vi "GetDigital.vi"(0 "reference in":refnum<class "Digital.lvclass">, 5 "error in (no error)":errorcluster) -> (14 "reference out":refnum<class "Digital.lvclass">, 19 "error out":errorcluster)   [LabVIEW 2019, in "Digital.lvclass"]
doc: "Draws A button"
uses:
  Digital.lvclass
  C:/Users/Taylor.Hillegeist/OneDrive - Ultra/LabVIEW/Pgui2/Pgui_Obj_class/Pgui_Obj.lvclass
  Pgui_Obj_class/Pgui_Obj.lvclass
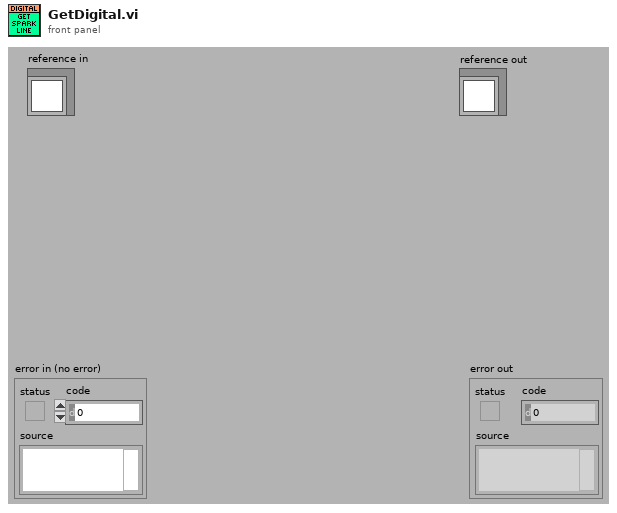
[diagram p1: front panel]
types:
  T1 = cluster{"left":i16, "top":i16, "right":i16, "bottom":i16}
  T2 = typedef "Digital.lvclass/ObjectAttributes.ctl" = cluster{"Override size":cluster{"Width":i16, "Height":i16}, "Value":dbl, "Digits Total":dbl, "Digits Precision":dbl}
  T3 = typedef "Pgui_Obj.lvclass/ObjectAttributes.ctl" = cluster{"Children":refnum<class "Pgui_Obj.lvclass">[], "Draw Instr":picture, "Params":cluster{"left":i16, "top":i16, "right":i16, "bottom":i16}, "Parent_Pgui_Obj":refnum<class "Pgui_Obj.lvclass">, "MouseOver":bool}
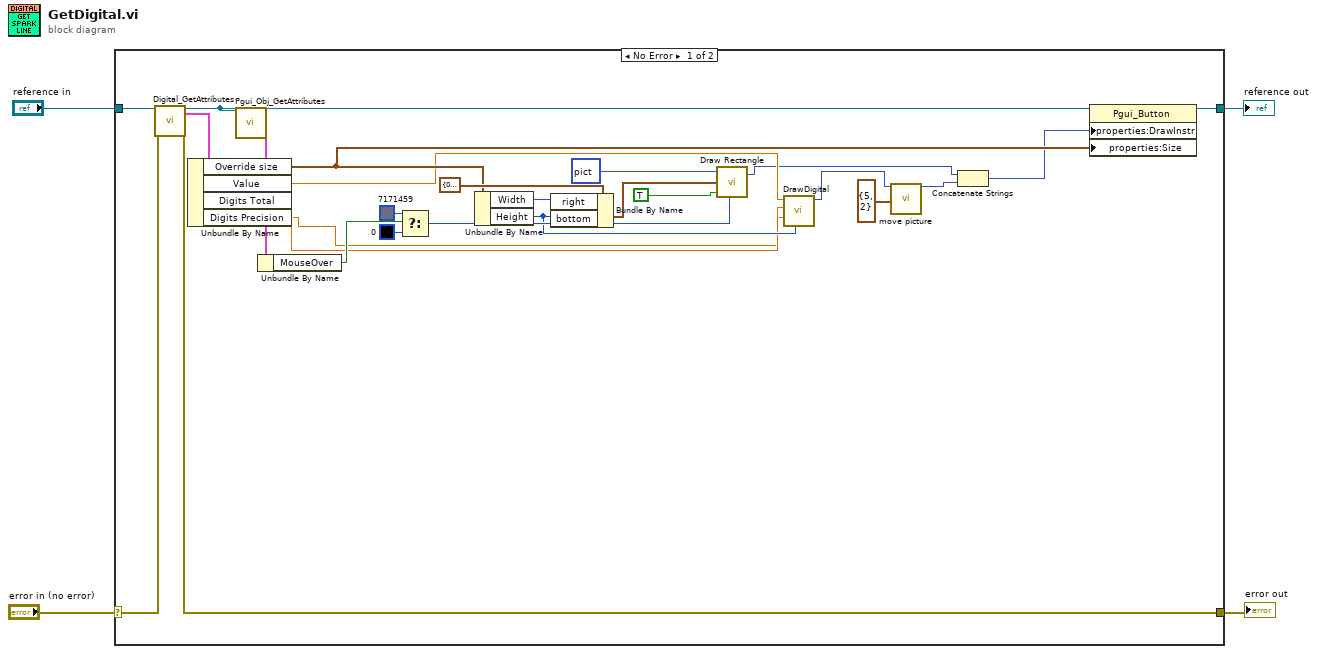
[diagram p0: block diagram]
diagram:
  n1 = case shown="No Error" "error in (no error)" {
    selector: "error in (no error)" -> [w30 w32]
    tunnel: [w28 w32] -> w3
    tunnel: [w24 w31] -> w1
    tunnel: "reference in" -> [w27 w31]
    frame No Error {
      n2 = call "Digital_GetAttributes.vi"("reference in"=w27, "error in (no error)"=w30) -> ("reference out"=w26:refnum<class "Digital.lvclass">, "Data"=w29:T2, "error out"=w28:errorcluster)  [unwired: 14 in, 1 out]
      n3 = Unbundle By Name(w29) -> ("Override size"=w14:cluster{"Width":i16, "Height":i16}, "Value"=w10:dbl, "Digits Total"=w12:dbl, "Digits Precision"=w11:dbl)
      n4 = call "Pgui_Obj_GetAttributes.vi"("reference in"=w26) -> ("Data"=w25:T3)  [unwired: 15 in, 3 out]
      n5 = Unbundle By Name(w25) -> ("MouseOver"=w15:bool)
      n6 = Select(t=u32 7171459 ("BG color(transparent)"), s=w15, f=u32 0 ("BG color(transparent)")) -> (s? t:f=w20:u32)
      n7 = Unbundle By Name(w14) -> ("Width"=w16:i16, "Height"=w13:i16)
      n8 = Bundle By Name(cluster=T1 {"left"=0, "top"=0, "right"=0, "bottom"=0} ("rect"), "right"=w16, "bottom"=w13) -> (w17:T1)
      n9 = call <vilib>:"Draw Rectangle.vi"("picture"=picture data[5B], "rect"=w17, "fill?(F)"=TRUE, "color(black)"=w20) -> ("new picture"=w6:picture)  [unwired: 5 in]
      n10 = call "DrawDigital.vi"("TextHeight"=w13, "precision (2)"=w11, "width (5)"=w12, "Value"=w10) -> ("Digital Display"=w9:picture)  [unwired: 7 in]
      n11 = call "move picture.vi"("Picture in"=w9, "move"=cluster{"x":i16, "y":i16} {"x"=5, "y"=2}) -> ("Picture out"=w7:picture)  [unwired: 17 in]
      n12 = Concatenate Strings(w6, w7) -> (w5:picture)
      n13 = property class="Pgui_Button"(reference=w26, "properties:DrawInstr"=w5, "properties:Size"=w14) -> (reference out=w24:refnum<class "Digital.lvclass">)  [unwired: 1 in, 1 out]
    }
    frame Error {
    }
  }
  "error out" <- w3
  "reference out" <- w1
